vi "Dashboard Main.vi"() -> ()   [LabVIEW 2013]
uses:
  <vilib>/Rock Robotics/WPI/Camera/WPI_CameraSettings Read MJPG.ctl
  <vilib>/Rock Robotics/WPI/Camera/WPI_CameraImageSize.ctl
  <vilib>/event_ctls.llb/eventvkey.ctl
panel:
  out "Ready To Fire":bool
  out "Catapult Clear":bool
  out "Puncher Clear":bool
  out "Roller Clear":bool
  out "high gear with words":enum16{"High Gear", "Low Gear"}(ring)
  out "High Gear":bool
  in  "Rec Mode":enum32{"Stop", "Record", "Playback"}(radio)
  out "Battery":sgl
  out "Speed":dbl(knob) scale=-25.0..25.0
  out "Dashboard Connected":bool
  in  "Tab Control":T1(tab)
  in  "New autonmous program":bool
  in  "Autonmous To Run":string(combo)
  in  "Autonmous mode":string
  in  "Editable":bool
  in  "Reload Autonmous text file":bool
  in  "Save Auto file back to text file":bool
  in  "Reload Constants":bool
  out "Variable Names":string[](array[string])
  out "Array of Numbers":dbl[](array[numeric])
  in  "Listbox":i32(listbox)
  in  "Stop Dashboard vision":bool
  in  "Enable vision":bool
  out "Camera":T2(plugin-control)
  out "Camera IP":string
  in  "Reset Gyro":bool
  out "gyroAngle":dbl
  out "Encoder Speed":dbl(graph)
  out "Second Catapult Limit":bool
  out "First Catapult Limit":bool
  in  "Gyro":bool
  in  "Encoder":bool
  out "Gyro Angle":dbl
  out "Encoder distance":dbl
  in  "Catapult test":bool
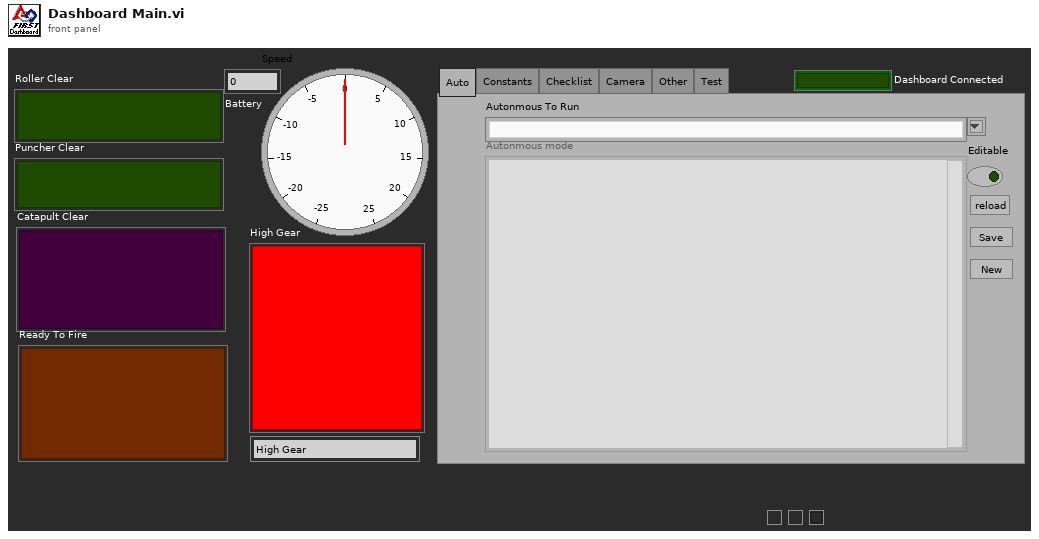
[diagram p1: front panel]
types:
  T1 = enum32{"Auto", "Constants", "Checklist", "Camera", "Other", "Test"}
  T2 = typedef "IMAQ Image.ctl" = refnum<image>
  T3 = typedef "Image Type" = u32
  T4 = enum16{"None", "On Hover", "On Key Focus", "On Hover or Key Focus"}
  T5 = enum8{"Enabled", "Disabled", "Disabled and Grayed Out"}
  T6 = cluster{"Digital Inputs":bool[], "Digital Outputs":bool[]}
  T7 = cluster{"Competition mode":bool, "Robot Link":bool, "Autonomous":bool, "Enabled":bool, "E-Stop":bool, "Simulated":bool, "TestMode":bool, "Docked Window":bool}
  T8 = typedef "WPI_CameraSettings Read MJPG.ctl" = cluster{"fps":i32, "compression":i32, "Image Size":T9}
  T9 = typedef "WPI_CameraImageSize.ctl" = enum16{"640x480", "320x240", "160x120"}
  T10 = cluster{cluster{dbl, dbl}, cluster{dbl, dbl}, cluster{dbl, dbl}}
  T11 = typedef "eventvkey.ctl" = enum16{"ASCII", "Enter", "Return", "Shift", "Ctrl", "Alt", "Cmd", "Opt", "Caps", "NumLock", "Clear", "Break", "Up", "Down", "Left", "Right", "Insert", "Delete", "Home", "End", "PageUp", "PageDown", "Escape", "Help", "Pause", "ScrollLock", "F1", "F2", "F3", "F4", "F5", "F6", "F7", "F8", "F9", "F10", "F11", "F12", "F13", "F14", "F15", "F16", "F17", "F18", "F19", "F20", "F21", "F22", "F23", "F24", "Play", "VolumeUp", "VolumeDown", "Mute", "Two Byte Char"}
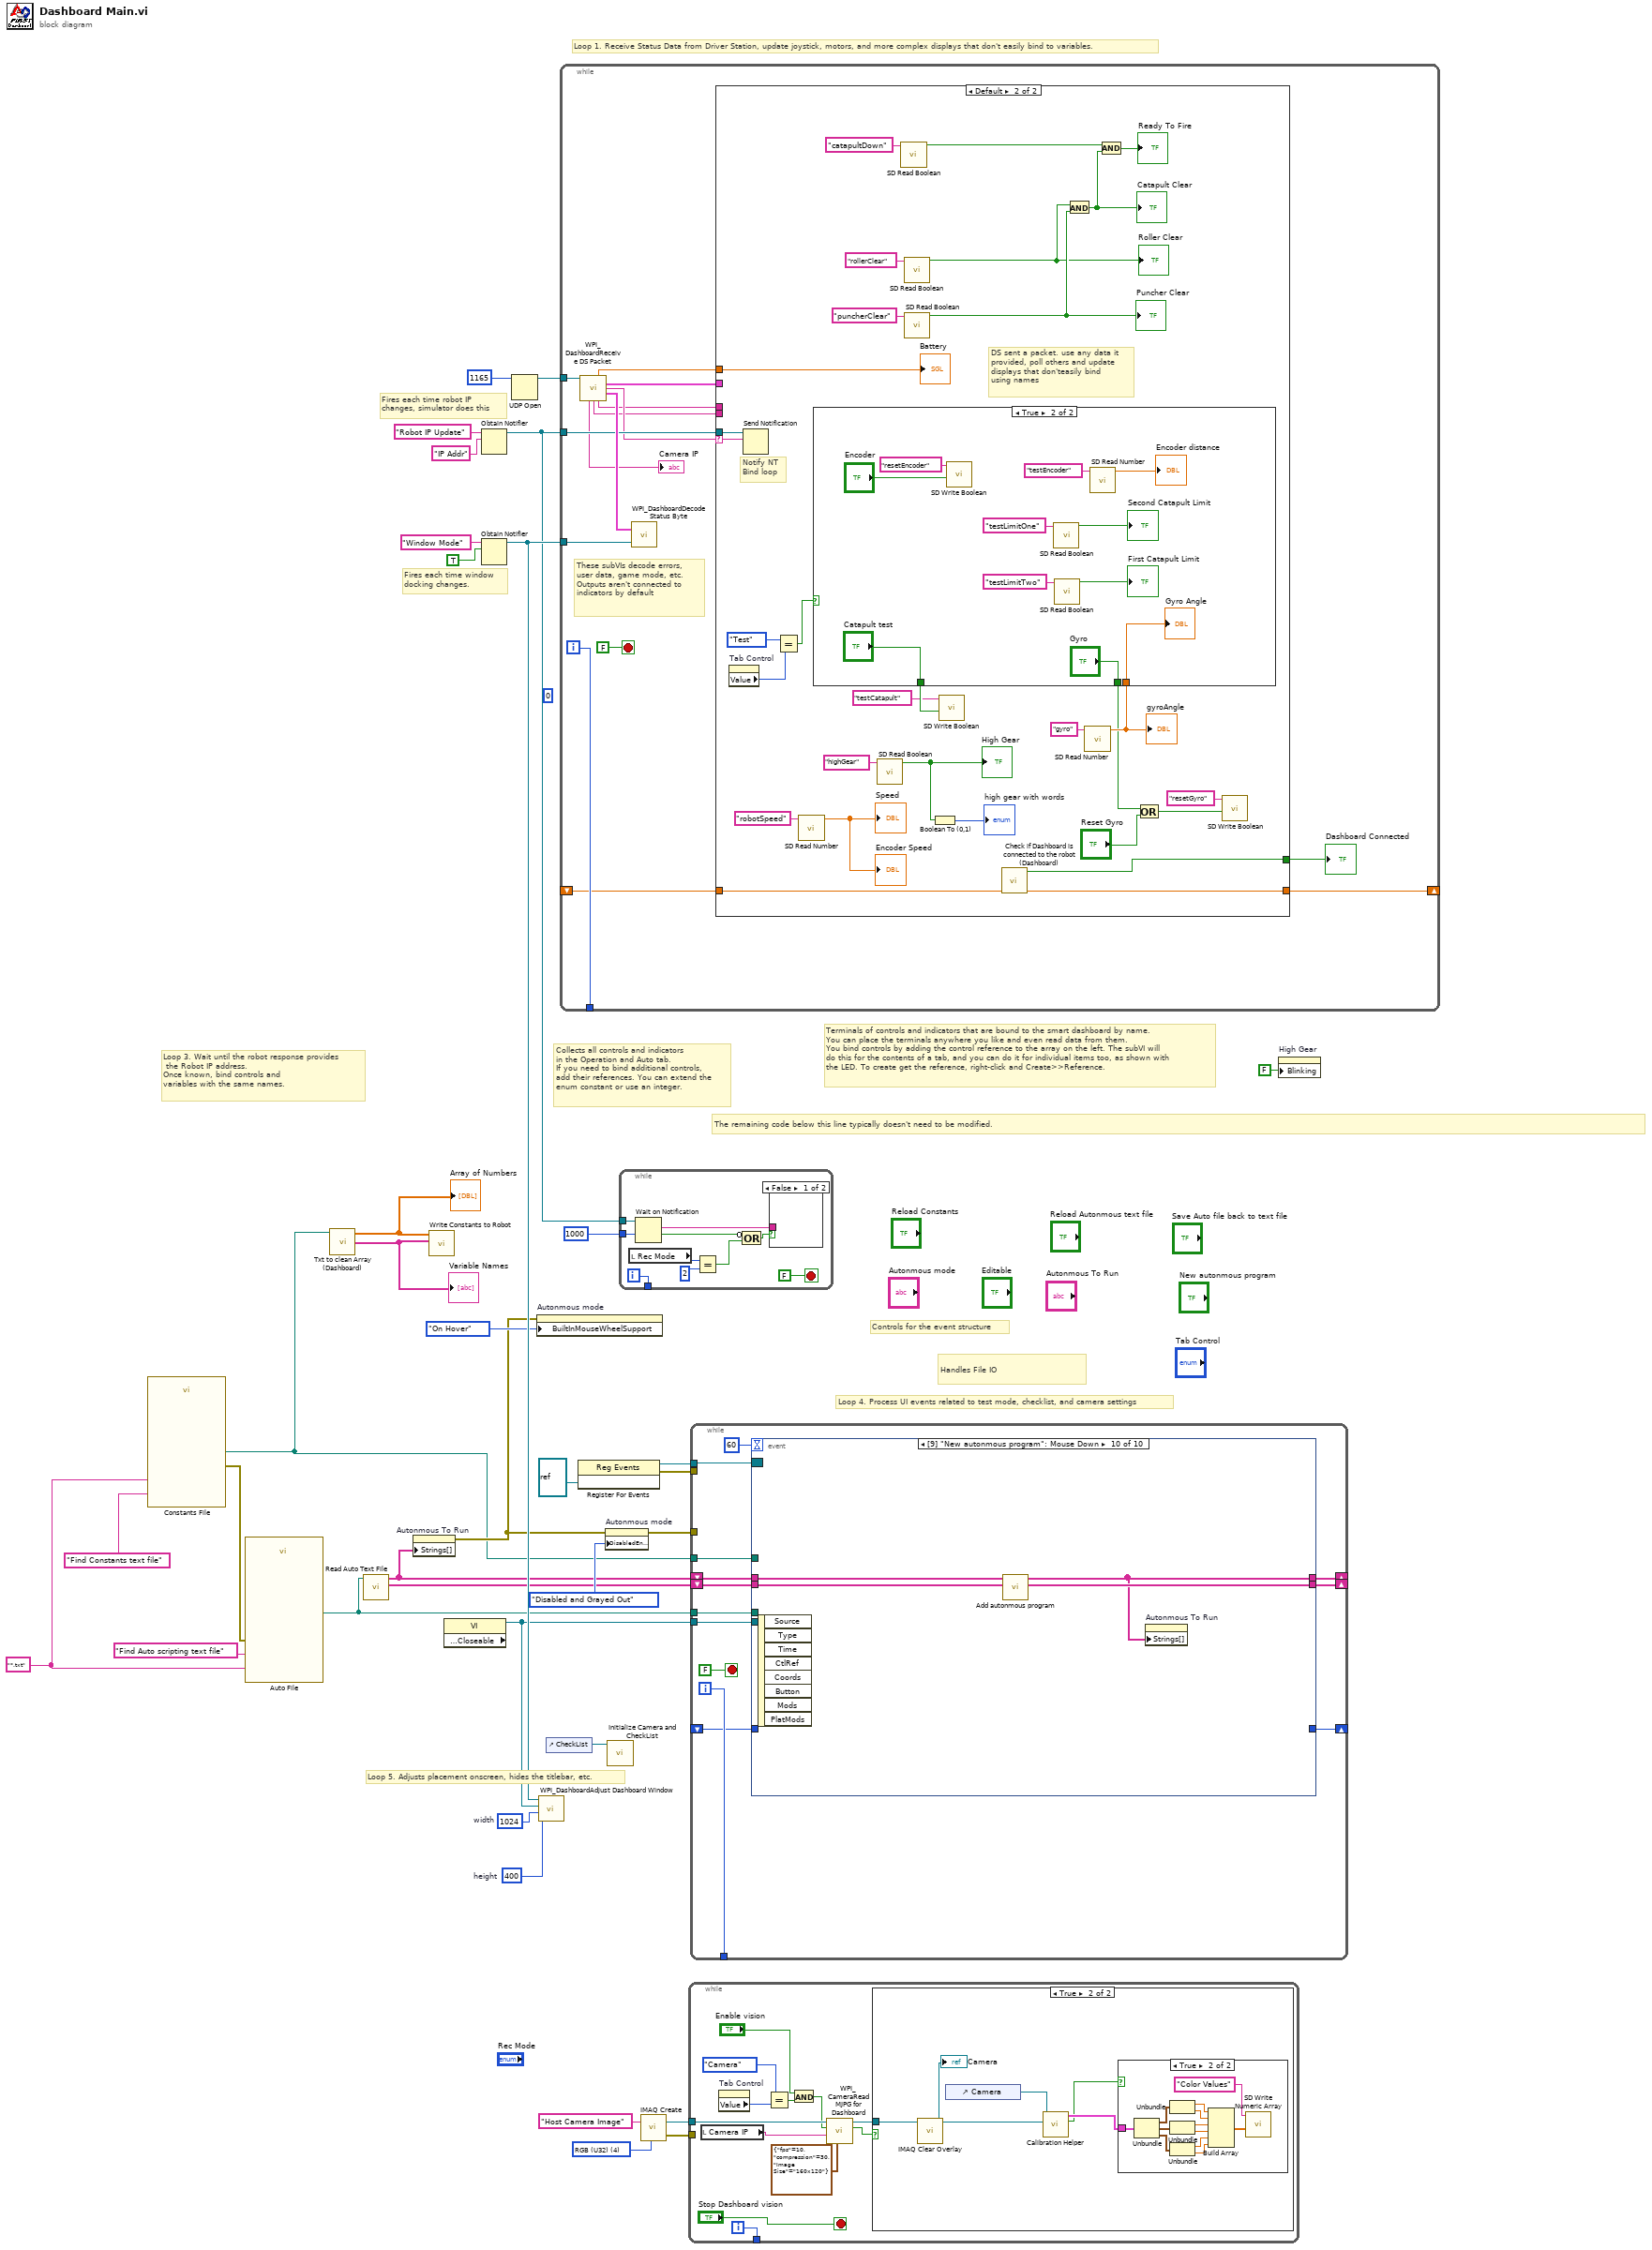
[diagram p0: block diagram]
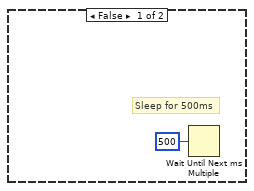
[diagram p2: hidden frame]
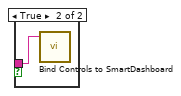
[diagram p4: hidden frame]
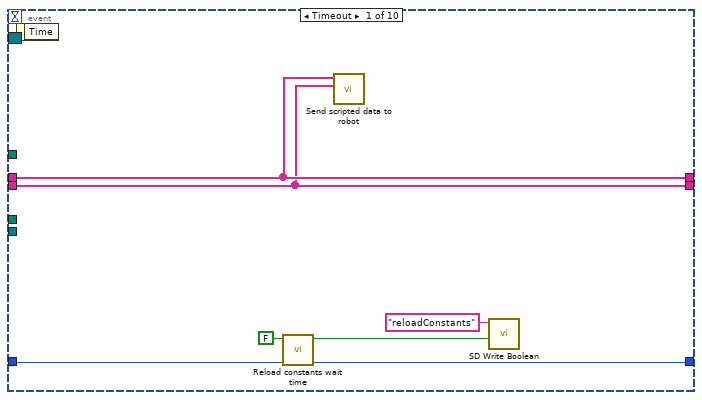
[diagram p5: hidden frame]
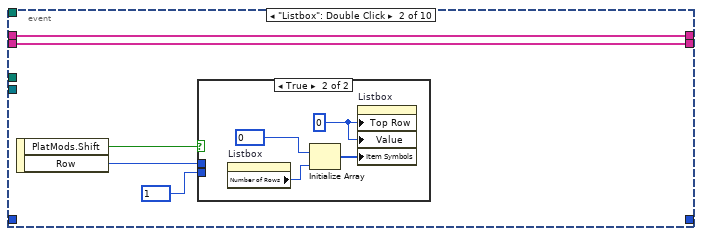
[diagram p6: hidden frame]
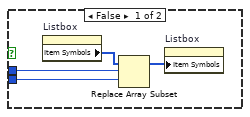
[diagram p7: hidden frame]
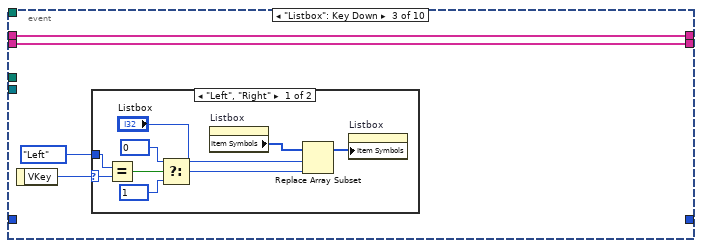
[diagram p8: hidden frame]
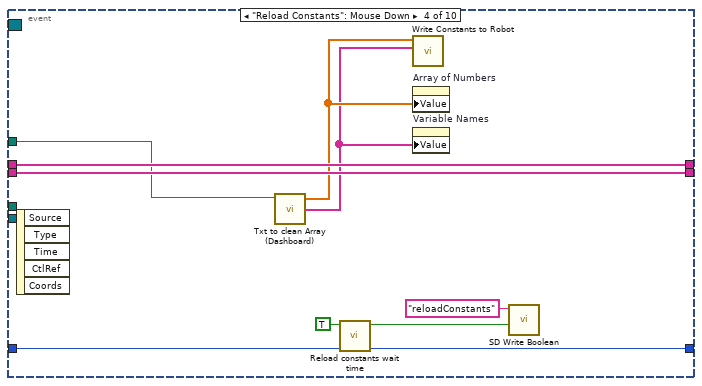
[diagram p10: hidden frame]
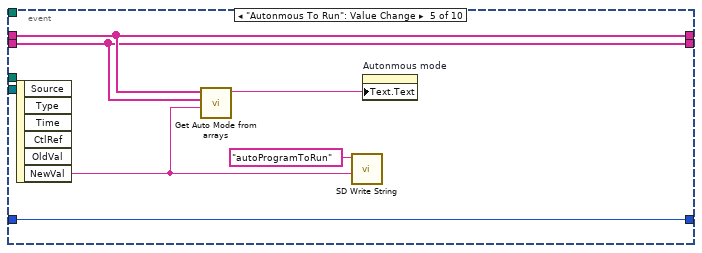
[diagram p11: hidden frame]
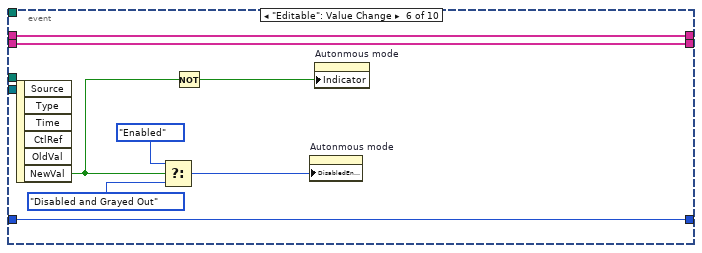
[diagram p12: hidden frame]
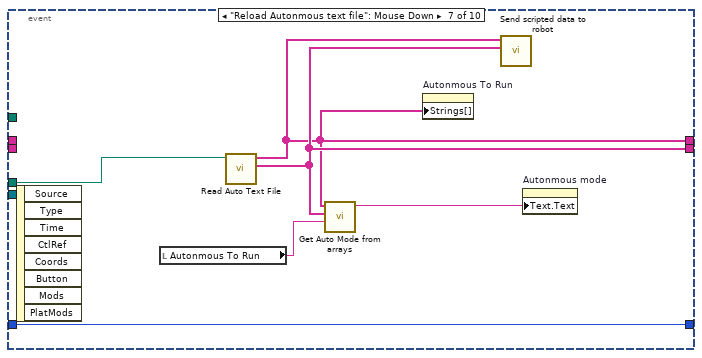
[diagram p13: hidden frame]
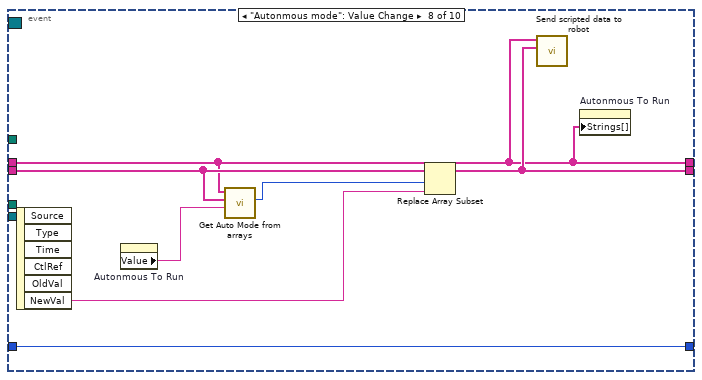
[diagram p14: hidden frame]
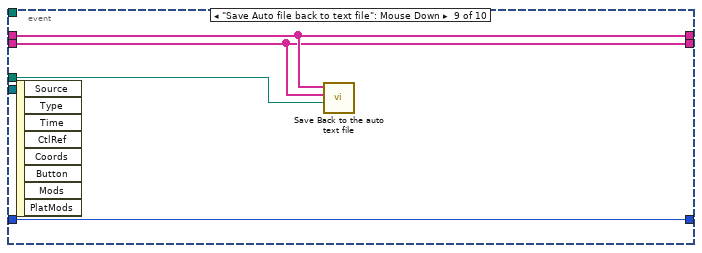
[diagram p15: hidden frame]
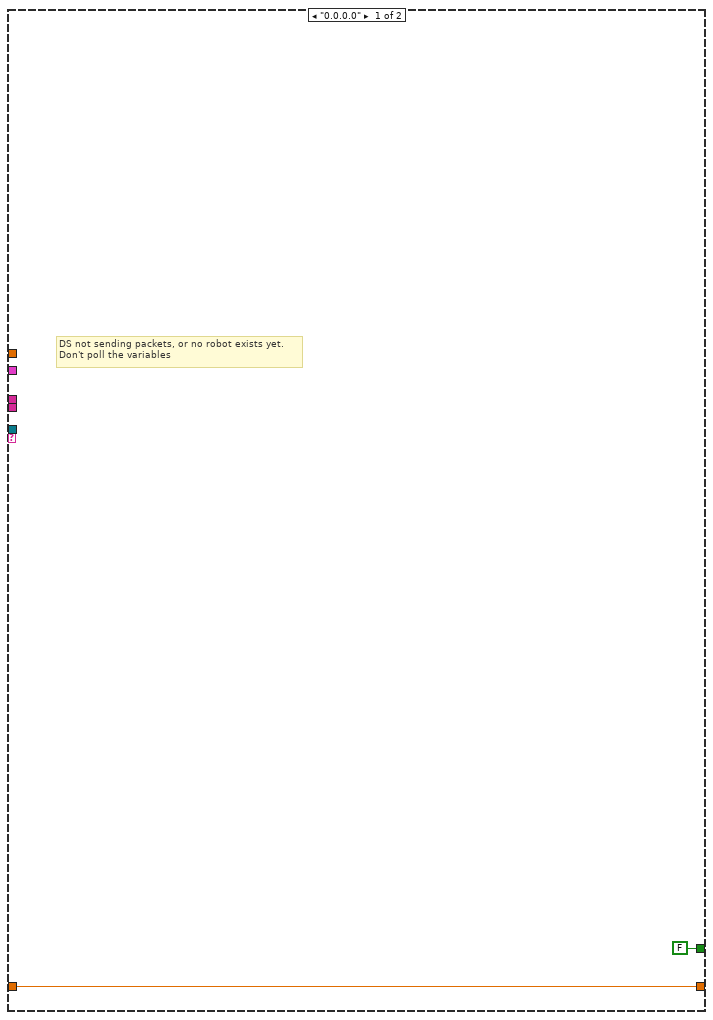
[diagram p16: hidden frame]
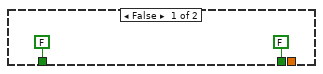
[diagram p17: hidden frame]
diagram:
  w4 = T3 4 items=["Grayscale (U8)", "Grayscale (I16)", "Grayscale (SGL)", "Complex (CSG)", "RGB (U32)", "HSL (U32)", "RGB (U64)"] ("Image Type")
  (unwired) u32 0 ("millisecond timer value out")
  w11 = "*.txt" ("pattern label")
  w25 = 400  # height
  w26 = 1024  # width
  # "Loop 3. Wait until the robot response provides\n the Robot IP address.\nOnce known, bind controls and\nvariables with the same names."
  # "Controls for the event structure"
  # "Handles File IO"
  # "Fires each time robot IP\nchanges, simulator does this"
  # "Fires each time window\ndocking changes."
  # "Collects all controls and indicators\nin the Operation and Auto tab.\nIf you need to bind additional controls,\nadd their references. You can extend the\nenum constant or use an integer."
  # "The remaining code below this line typically doesn't need to be modified."
  # "Loop 4. Process UI events related to test mode, checklist, and camera settings"
  # "Terminals of controls and indicators that are bound to the smart dashboard by name.\nYou can place the terminals anywhere you like and even read data from them.\nYou bind controls by adding the control reference to the array on the left. The subVI will\ndo this for the contents of a tab, and you can do it for individual items too, as shown with\nthe LED. To create get the reference, right-click and Create>>Reference."
  # "Loop 5. Adjusts placement onscreen, hides the titlebar, etc."
  # "Loop 1. Receive Status Data from Driver Station, update joystick, motors, and more complex displays that don't easily bind to variables."
  n1 = call "Constants File"("prompt"="Find Constants text file", "pattern (all files)"=w11) -> ("selected path"=w14:path, "error out"=w13:errorcluster)  [unwired: 10 in, 2 out]
  n2 = call "Auto File"("prompt"="Find Auto scripting text file", "error in"=w13, "pattern (all files)"=w11) -> ("selected path"=w21:path)  [unwired: 9 in, 3 out]
  n3 = call "Txt to clean Array (Dashboard).vi"("file path"=w14) -> ("Variable Names"=w8:string[], "Array of Numbers"=w9:dbl[])  [unwired: 3 in, 1 out]
  "Array of Numbers" <- w9
  "Variable Names" <- w8
  n4 = call "Read Auto Text File.vi"("selected path"=w21) -> ("Programs"=w18:string[], "Program Name"=w19:string[])  [unwired: 8 in, 1 out]
  n5 = property on="Autonmous To Run" class="CmbBox"("Strings[]"=w19) -> (error out=w16:errorcluster)  [unwired: 2 in, 1 out]
  n6 = call "Write Constants to Robot.vi"("Variable Names"=w8, "Array of Numbers"=w9) -> ()  [unwired: 10 in]
  n7 = property class="VI" props=["Front Panel.Closeable"]() -> (reference out=w22:refnum<vi>)  [unwired: 2 in, 2 out]
  n8 = Obtain Notifier(name (unnamed)="Robot IP Update", notification data type="IP Addr" ("name (unnamed)")) -> (notifier out=w5:refnum<notifier>)  [unwired: 2 in, 2 out]
  n9 = Obtain Notifier(name (unnamed)="Window Mode", notification data type=TRUE) -> (notifier out=w24:refnum<notifier>)  [unwired: 2 in, 2 out]
  n10 = UDP Open(11:u16 1165 ("port")) -> (port=w34:refnum<k16>)  [unwired: 2 in, 4 out]
  n11 = property on="Autonmous mode" class="Str"(error in=w16, "BuiltInMouseWheelSupport"=T4."On Hover" ("Built-In Mouse Wheel Support")) -> ()  [unwired: 1 in, 2 out]
  n12 = call <vilib>:"WPI_DashboardAdjust Dashboard Window.vi"("height"=w25, "width"=w26, "reference in"=w22, "Notifier in"=w24) -> ()  [unwired: 8 in]
  n13 = control-ref of="CheckList"() -> (w23:refnum<vi>)
  n14 = while {
    tunnel: w34 -> [w48]
    tunnel: w5 -> [w45]
    tunnel: w24 -> [w47]
    tunnel: [w46] -> _
    shift-right: [w39] -> _
    shift-left: _ -> [w38]
    i -> [w46]
    stop <- FALSE stop-if-true
    # "These subVIs decode errors, user data, game mode, etc.\nOutputs aren't connected to indicators by default"
    n15 = call <vilib>:"WPI_DashboardReceive DS Packet.vi"("Recv Socket"=w48) -> ("Battery"=w40:sgl, "Driver Station"=w41:T6, "Robot IP Address"=w44:string, "Status"=w49:T7, "Camera IP Address"=→"Camera IP":string, "Low Priority User Data"=w43:string, "High Priority User Data"=w42:string)  [unwired: 1 in, 7 out]
    n16 = call <vilib>:"WPI_DashboardDecode Status Byte.vi"("Window Mode Notifier"=w47, "Status"=w49) -> ()  [unwired: 2 out]
    n17 = case shown="Default" w44 {
      selector: w44 -> [_ w81]
      tunnel: w45 -> [_ w82]
      tunnel: w43 -> [_ _]
      tunnel: w42 -> [_ _]
      tunnel: w41 -> [_ _]
      tunnel: w40 -> [_ w76]
      tunnel: [w52 w80] -> w39
      tunnel: w38 -> [w52 w79]
      tunnel: [FALSE ("Number Changing") w75] -> w37
      frame "0.0.0.0" {
        # "DS not sending packets, or no robot exists yet.\nDon't poll the variables"
      }
      frame Default {
        # "Notify NT\nBind loop"
        # "DS sent a packet. use any data it\nprovided, poll others and update\ndisplays that don'teasily bind\nusing names"
        n18 = property on="Tab Control" class="TabCtl (strict)"() -> ("Value"=w69:T1)  [unwired: 2 in, 2 out]
        n19 = Send Notification(notification=w81, notifier=w82) -> ()  [unwired: 1 in, 2 out]
        n20 = Equal?(x=T1."Test", y=w69) -> (x = y?=w67:bool)
        n21 = call <vilib>:"SD Read Number.vi"("Name"="robotSpeed") -> ("Numeric"=→"Speed" →"Encoder Speed":dbl)  [unwired: 8 in, 2 out]
        n22 = call <vilib>:"SD Read Boolean.vi"("Name"="highGear") -> ("Boolean"=w71:bool)  [unwired: 8 in, 2 out]
        "High Gear" <- w71
        n23 = call <vilib>:"SD Read Boolean.vi"("Name"="catapultDown") -> ("Boolean"=w54:bool)  [unwired: 8 in, 2 out]
        n24 = call <vilib>:"SD Read Boolean.vi"("Name"="rollerClear") -> ("Boolean"=w56:bool)  [unwired: 8 in, 2 out]
        "Roller Clear" <- w56
        n25 = call <vilib>:"SD Read Boolean.vi"("Name"="puncherClear") -> ("Boolean"=w57:bool)  [unwired: 8 in, 2 out]
        "Puncher Clear" <- w57
        n26 = Boolean To (0,1)(Boolean=w71) -> (0, 1=→"high gear with words":i16)
        n27 = call "Check if Dashboard is connected to the robot (Dashboard).vi"("From shift"=w79) -> ("to shift"=w80:dbl, "Number Changing"=w75:bool)  [unwired: 9 in]
        n28 = And(x=w56, y=w57) -> (x .and. y?=w55:bool)
        "Catapult Clear" <- w55
        n29 = call <vilib>:"SD Read Number.vi"("Name"="gyro") -> ("Numeric"=w64:dbl)  [unwired: 8 in, 2 out]
        "gyroAngle" <- w64
        n30 = case shown="True" w67 {
          tunnel: w64 -> [_ w95]
          tunnel: [FALSE ("Gyro") "Gyro"] -> w63
          tunnel: [FALSE ("Catapult test") "Catapult test"] -> w62
          frame False {
          }
          frame True {
            n31 = call <vilib>:"SD Write Boolean.vi"("Boolean"="Encoder", "Name"="resetEncoder") -> ()  [unwired: 8 in, 2 out]
            n32 = call <vilib>:"SD Read Boolean.vi"("Name"="testLimitOne") -> ("Boolean"=→"Second Catapult Limit":bool)  [unwired: 8 in, 2 out]
            n33 = call <vilib>:"SD Read Boolean.vi"("Name"="testLimitTwo") -> ("Boolean"=→"First Catapult Limit":bool)  [unwired: 8 in, 2 out]
            n34 = call <vilib>:"SD Read Number.vi"("Name"="testEncoder") -> ("Numeric"=→"Encoder distance":dbl)  [unwired: 8 in, 2 out]
            "Gyro Angle" <- w95
          }
        }
        n35 = call <vilib>:"SD Write Boolean.vi"("Boolean"=w62, "Name"="testCatapult") -> ()  [unwired: 8 in, 2 out]
        n36 = And(x=w54, y=w55) -> (x .and. y?=→"Ready To Fire":bool)
        n37 = Or(x=w63, y="Reset Gyro") -> (x .or. y?=w65:bool)
        n38 = call <vilib>:"SD Write Boolean.vi"("Boolean"=w65, "Name"="resetGyro") -> ()  [unwired: 8 in, 2 out]
        "Battery" <- w76
      }
    }
    "Dashboard Connected" <- w37
  }
  n39 = register-events(refnum<vi> refnum) -> (reference out=w29:refnum<event-registration>, error out=w28:errorcluster)  [unwired: 2 in]
  n40 = property on="Autonmous mode" class="Str"(error in=w16, "DisabledEnum"=T5."Disabled and Grayed Out" ("Disabled")) -> (error out=w15:errorcluster)  [unwired: 1 in, 1 out]
  n41 = call "Initialize Camera and CheckList.vi"("ListBox in"=w23) -> ()  [unwired: 11 in]
  n42 = while {
    tunnel: w5 -> [w104]
    tunnel: [w102] -> _
    tunnel: u32 1000 ("milliseconds to wait") -> [w101]
    i -> [w102]
    stop <- FALSE stop-if-true
    n43 = local read "Rec Mode"() -> (w97:enum32{"Stop", "Record", "Playback"})
    n44 = Wait on Notification(notifier=w104, timeout in ms (-1)=w101) -> (notification=w103:string, timed out?=w99:bool)  [unwired: 2 in, 2 out]
    n45 = Equal?(x=w97, y=u16 2 ("Rec Mode")) -> (x = y?=w98:bool)
    n46 = Compound Arithmetic op=OR(invert w99, w98) -> (w100:bool)
    n47 = case shown="False" w100 {
      tunnel: w103 -> [_ w106]
      frame False {
      }
      frame True {
        n48 = call <vilib>:"Bind Controls to SmartDashboard.vi"("Server IP Address"=w106) -> ()  [unwired: 11 in]
      }
    }
  }
  n49 = call "IMAQ Create"("Image Name"="Host Camera Image", "Image Type"=w4) -> ("New Image"=w2:T2, "error out"=w1:errorcluster)  [unwired: 2 in, 1 out]
  n50 = while {
    tunnel: w2 -> [w117]
    tunnel: [w118] -> _
    tunnel: w1 -> [_]
    i -> [w118]
    stop <- "Stop Dashboard vision" stop-if-true
    n51 = local read "Camera IP"() -> (w113:string)
    n52 = property on="Tab Control" class="TabCtl (strict)"() -> ("Value"=w112:T1)  [unwired: 2 in, 2 out]
    n53 = Equal?(x=T1."Camera", y=w112) -> (x = y?=w111:bool)
    n54 = And(x="Enable vision", y=w111) -> (x .and. y?=w109:bool)
    n55 = call <vilib>:"WPI_CameraRead MJPG for Dashboard.vi"("Camera Settings"=T8 {"fps"=10, "compression"=30, "Image Size"=enum."160x120"}, "Camera IP"=w113, "Enable"=w109, "Refnum in"=w117) -> ("Active"=w115:bool, "Refnum out"=w116:T2)  [unwired: 4 in, 2 out]
    n56 = case shown="True" w115 {
      tunnel: w116 -> [_ w120]
      frame False {
        # "Sleep for 500ms"
        n57 = Wait Until Next ms Multiple(millisecond multiple=u32 500) -> ()  [unwired: 1 out]
      }
      frame True {
        n58 = call "IMAQ Clear Overlay"("Image"=w120) -> ("Image Out"=w121:T2)  [unwired: 9 in, 1 out]
        "Camera" <- w121
        n59 = control-ref of="Camera"() -> (w122:refnum<vi>)
        n60 = call "Calibration Helper.vi"("Image"=w121, "Image Ctl Refnum"=w122) -> ("Changed"=w123:bool, "output color"=w124:T10)  [unwired: 8 in]
        n61 = case shown="True" w123 {
          tunnel: w124 -> [_ w125]
          frame False {
          }
          frame True {
            n62 = Unbundle(w125) -> (w134:cluster{dbl, dbl}, w136:cluster{dbl, dbl}, w135:cluster{dbl, dbl})
            n63 = Unbundle(w134) -> (w133:dbl, w132:dbl)
            n64 = Unbundle(w136) -> (w131:dbl, w130:dbl)
            n65 = Unbundle(w135) -> (w129:dbl, w128:dbl)
            n66 = Build Array(w133, w132, w131, w130, w129, w128) -> (w127:dbl[])
            n67 = call <vilib>:"SD Write Numeric Array.vi"("Numeric Array"=w127, "Name"="Color Values") -> ()  [unwired: 8 in, 2 out]
          }
        }
      }
    }
  }
  n68 = while {
    tunnel: [w147] -> _
    tunnel: w29 -> [w146]
    tunnel: w28 -> [_]
    tunnel: w22 -> [w145]
    tunnel: w21 -> [w144]
    tunnel: w14 -> [w143]
    shift-right: [w140] -> _
    shift-left: w19 -> [w142]
    shift-right: [w139] -> _
    shift-left: w18 -> [w141]
    tunnel: w15 -> [_]
    shift-right: [w138] -> _
    shift-left: _ -> [w137]
    i -> [w147]
    stop <- FALSE stop-if-true
    n69 = event shown="[9] \"New autonmous program\": Mouse Down" {
      selector: w146 -> [_ _ _ _ _ _ _ _ _ _]
      dyn-events: _ -> [_ _ _ _ _ _ _ _ _ _]
      timeout: u32 60 ("milliseconds to wait") -> [_ _ _ _ _ _ _ _ _ _]
      tunnel: w145 -> [_ _ _ _ _ _ _ _ _ _]
      tunnel: w144 -> [_ _ _ _ _ _ w212 _ w221 _]
      tunnel: w143 -> [_ _ _ w190 _ _ _ _ _ _]
      tunnel: w141 -> [w155 w157 w170 w191 w194 w200 _ w218 w222 w226]
      tunnel: w142 -> [w156 w158 w171 w192 w195 w201 _ w215 w223 w227]
      tunnel: [w156 w158 w171 w192 w195 w201 w208 w215 w223 w224] -> w140
      tunnel: [w155 w157 w170 w191 w194 w200 w211 w216 w222 w225] -> w139
      tunnel: [w153 _ _ w186 w193 w199 w207 w213 w220 _] -> w138
      tunnel: w137 -> [w154 _ _ w187 w193 w199 w207 w213 w220 _]
      event Timeout {
        n70 = event-data() -> ()  [unwired: 1 in, 1 out]
        n71 = call "Reload constants wait time.vi"("millisecond timer value in"=w154, "Reload Constants"=FALSE) -> ("millisecond timer value out"=w153:u32, "Tell Robot to reload constants"=w150:bool)  [unwired: 8 in]
        n72 = call "Send scripted data to robot.vi"("Programs"=w155, "Program Name"=w156) -> ()  [unwired: 10 in]
        n73 = call <vilib>:"SD Write Boolean.vi"("Boolean"=w150, "Name"="reloadConstants") -> ()  [unwired: 8 in, 2 out]
      }
      event "Listbox": Double Click {
        n74 = event-data() -> ("PlatMods.Shift"=w159:bool, "Row"=w161:i32)  [unwired: 1 in]
        n75 = case shown="True" w159 {
          tunnel: w161 -> [w165 _]
          tunnel: 1 -> [w164 _]
          frame False {
            n76 = property on="Listbox" class="LstBox (strict)"() -> ("Item Symbols"=w163:i32[])  [unwired: 2 in, 2 out]
            n77 = Replace Array Subset(array=w163, new element=w164, index=w165) -> (w162:i32[])
            n78 = property on="Listbox" class="LstBox (strict)"("Item Symbols"=w162) -> ()  [unwired: 2 in, 2 out]
          }
          frame True {
            w166 = 0 ("Top Row")
            n79 = property on="Listbox" class="LstBox (strict)"() -> ("Number of Rows"=w168:u32)  [unwired: 2 in, 2 out]
            n80 = Initialize Array(0, w168) -> (w167:i32[])
            n81 = property on="Listbox" class="LstBox (strict)"("Top Row"=w166, "Value"=w166, "Item Symbols"=w167) -> ()  [unwired: 2 in, 2 out]
          }
        }
      }
      event "Listbox": Key Down {
        n82 = event-data() -> ("VKey"=w173:T11)  [unwired: 1 in]
        n83 = case shown="\"Left\", \"Right\"" w173 {
          selector: w173 -> [w178 _]
          tunnel: eventvkey."Left" ("VKey") -> [w176 _]
          frame "Left", "Right" {
            n84 = Equal?(x=w176, y=w178) -> (x = y?=w177:bool)
            n85 = Select(t=0, s=w177, f=1) -> (s? t:f=w179:i32)
            n86 = property on="Listbox" class="LstBox (strict)"() -> ("Item Symbols"=w182:i32[])  [unwired: 2 in, 2 out]
            n87 = Replace Array Subset(array=w182, new element=w179, index="Listbox") -> (w181:i32[])
            n88 = property on="Listbox" class="LstBox (strict)"("Item Symbols"=w181) -> ()  [unwired: 2 in, 2 out]
          }
          frame Default {
          }
        }
      }
      event "Reload Constants": Mouse Down {
        n89 = event-data() -> ()  [unwired: 1 in, 5 out]
        n90 = call "Txt to clean Array (Dashboard).vi"("file path"=w190) -> ("Variable Names"=w188:string[], "Array of Numbers"=w189:dbl[])  [unwired: 3 in, 1 out]
        n91 = call "Reload constants wait time.vi"("millisecond timer value in"=w187, "Reload Constants"=TRUE) -> ("millisecond timer value out"=w186:u32, "Tell Robot to reload constants"=w183:bool)  [unwired: 8 in]
        n92 = call "Write Constants to Robot.vi"("Variable Names"=w188, "Array of Numbers"=w189) -> ()  [unwired: 10 in]
        n93 = property on="Array of Numbers" class="Arr (strict)"("Value"=w189) -> ()  [unwired: 2 in, 2 out]
        n94 = property on="Variable Names" class="Arr (strict)"("Value"=w188) -> ()  [unwired: 2 in, 2 out]
        n95 = call <vilib>:"SD Write Boolean.vi"("Boolean"=w183, "Name"="reloadConstants") -> ()  [unwired: 8 in, 2 out]
      }
      event "Autonmous To Run": Value Change {
        n96 = event-data() -> ("NewVal"=w197:string)  [unwired: 1 in, 5 out]
        n97 = call "Get Auto Mode from arrays.vi"("Auto Name"=w197, "Programs"=w194, "Program Name"=w195) -> ("Auto Program"=w196:string)  [unwired: 7 in, 1 out]
        n98 = call <vilib>:"SD Write String.vi"("String"=w197, "Name"="autoProgramToRun") -> ()  [unwired: 8 in, 2 out]
        n99 = property on="Autonmous mode" class="Str"("Text.Text"=w196) -> ()  [unwired: 2 in, 2 out]
      }
      event "Editable": Value Change {
        n100 = event-data() -> ("NewVal"=w203:bool)  [unwired: 1 in, 5 out]
        n101 = Select(t=T5."Enabled" ("Disabled"), s=w203, f=T5."Disabled and Grayed Out" ("Disabled")) -> (s? t:f=w204:T5)
        n102 = Not(x=w203) -> (.not. x?=w202:bool)
        n103 = property on="Autonmous mode" class="Str"("DisabledEnum"=w204) -> ()  [unwired: 2 in, 2 out]
        n104 = property on="Autonmous mode" class="Str"("Indicator"=w202) -> ()  [unwired: 2 in, 2 out]
      }
      event "Reload Autonmous text file": Mouse Down {
        n105 = event-data() -> ()  [unwired: 1 in, 8 out]
        n106 = local read "Autonmous To Run"() -> (w210:string)
        n107 = call "Read Auto Text File.vi"("selected path"=w212) -> ("Programs"=w211:string[], "Program Name"=w208:string[])  [unwired: 8 in, 1 out]
        n108 = call "Get Auto Mode from arrays.vi"("Auto Name"=w210, "Programs"=w211, "Program Name"=w208) -> ("Auto Program"=w209:string)  [unwired: 7 in, 1 out]
        n109 = property on="Autonmous To Run" class="CmbBox"("Strings[]"=w208) -> ()  [unwired: 2 in, 2 out]
        n110 = call "Send scripted data to robot.vi"("Programs"=w211, "Program Name"=w208) -> ()  [unwired: 10 in]
        n111 = property on="Autonmous mode" class="Str"("Text.Text"=w209) -> ()  [unwired: 2 in, 2 out]
      }
      event "Autonmous mode": Value Change {
        n112 = event-data() -> ("NewVal"=w214:string)  [unwired: 1 in, 5 out]
        n113 = property on="Autonmous To Run" class="CmbBox"() -> ("Value"=w219:string)  [unwired: 2 in, 2 out]
        n114 = call "Get Auto Mode from arrays.vi"("Auto Name"=w219, "Programs"=w218, "Program Name"=w215) -> ("index"=w217:i32)  [unwired: 7 in, 1 out]
        n115 = Replace Array Subset(array=w218, new element=w214, index=w217) -> (w216:string[])
        n116 = call "Send scripted data to robot.vi"("Programs"=w216, "Program Name"=w215) -> ()  [unwired: 10 in]
        n117 = property on="Autonmous To Run" class="CmbBox"("Strings[]"=w215) -> ()  [unwired: 2 in, 2 out]
      }
      event "Save Auto file back to text file": Mouse Down {
        n118 = event-data() -> ()  [unwired: 1 in, 8 out]
        n119 = call "Save Back to the auto text file.vi"("Path"=w221, "Programs"=w222, "Program Name"=w223) -> ()  [unwired: 9 in]
      }
      event "New autonmous program": Mouse Down {
        n120 = event-data() -> ()  [unwired: 1 in, 8 out]
        n121 = call "Add autonmous program.vi"("Programs in"=w226, "Program Name in"=w227) -> ("Programs out"=w225:string[], "Program Name out"=w224:string[])  [unwired: 8 in]
        n122 = property on="Autonmous To Run" class="CmbBox"("Strings[]"=w224) -> ()  [unwired: 2 in, 2 out]
      }
    }
  }
  n123 = property on="High Gear" class="Bool (strict)"("Blinking"=FALSE) -> ()  [unwired: 2 in, 2 out]
